vi "CALC_FUNC_DATA.vi"(0 "VISA IN":refnum<visa-resource-name>, 5 "error in":errorcluster, 7 "Channel":i32) -> (14 "VISA Out":refnum<visa-resource-name>, 16 "Data":string, 19 "error out":errorcluster)   [LabVIEW 2018, in "PNA-X.lvlib"]
doc: "CALCulate<cnum>:FUNCtion:DATA? \n(Read-only) Returns the trace statistic data for the selected statistic type for the specified channel. \nSelect the type of statistic with CALC:FUNC:TYPE. \nSee Critical Note \nParameters \n<cnum> Channel number of the measurement. There must be a selected measurement on \nthat channel. If unspecified, <cnum> is set to 1. \nReturn Type Depends on FORM:DATA \nExample CALCulate2:FUNCtion:DATA? \nDefault Not applicable"
uses:
  PNA-X.lvlib
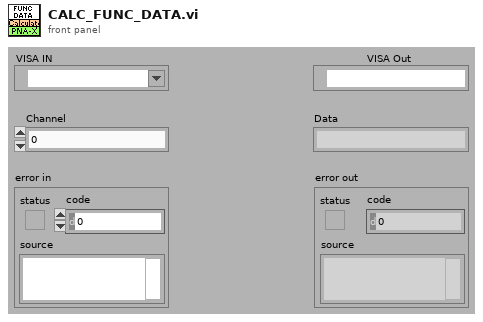
[diagram p1: front panel]
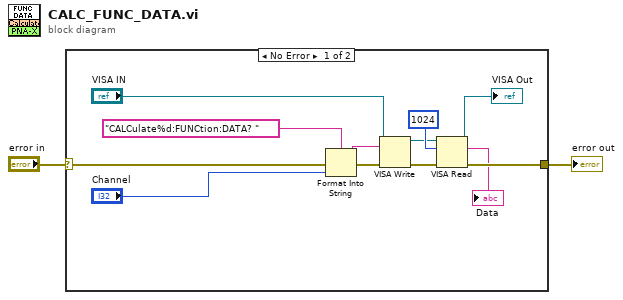
[diagram p0: block diagram]
diagram:
  n1 = case shown="No Error" "error in" {
    selector: "error in" -> [w14 w15]
    tunnel: [w6 w15] -> w1
    frame No Error {
      n2 = Format Into String(format string="CALCulate%d:FUNCtion:DATA? " ("Cmdline"), error in=w14, "Channel") -> (resulting string=w12:string, error out=w13:errorcluster)  [unwired: 1 in]
      n3 = VISA Write(VISA resource name="VISA IN", write buffer=w12, error in (no error)=w13) -> (VISA resource name out=w7:refnum<visa-resource-name>, error out=w9:errorcluster)  [unwired: 1 out]
      n4 = VISA Read(VISA resource name=w7, byte count=1024, error in (no error)=w9) -> (VISA resource name out=→"VISA Out":refnum<visa-resource-name>, read buffer=→"Data":string, error out=w6:errorcluster)  [unwired: 1 out]
    }
    frame Error {
    }
  }
  "error out" <- w1
